vi "LAChat.vi"   [LabVIEW 2017, in "LiteAgentSDK.lvlib"]
uses:
  LiteAgentSDK.lvlib
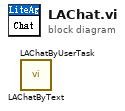
[diagram p0: block diagram]
diagram:
  n1 = call "LAChatByText.vi"() -> ()  [unwired: 10 in, 2 out]
  n2 = call "LAChatByUserTask.vi"() -> ()  [unwired: 10 in, 2 out]
